vi "DIO 1（Hsot）.vi"() -> ()   [LabVIEW 2019]
uses:
  <vilib>/FPGAPlugInAG/ELVIS III/niLvFpga_Open_ELVIS III.vi
  <vilib>/rvi/interface/common/dynamic/niFpgaDynamicAddResources.vi
  <vilib>/Utility/error.llb/Error Cluster From Error Code.vi
  <vilib>/rvi/errors/niLvFpgaAdjustHostInterfaceError.vi
  <vilib>/FPGAPlugInAG/Dynamic/niLvFpga_Close_Dynamic.vi
  <vilib>/rvi/interface/nirviOpenFPGA/nirviOpenFPGA.xnode
  FPGA Bitfiles/analogio-fpga_FPGATarget_DIO1_c7CcyW3shMY.lvbitx
  DIO 1.vi
  <vilib>/rvi/interface/nirviReadWriteControl/nirviReadWriteControl.xnode
  <vilib>/rvi/interface/nirviCloseFPGA/nirviCloseFPGA.xnode
  NiFpgaLv.dll
  <vilib>/rvi/interface/Simulation/niFpgaSimulationCallBeginRW.vi
panel:
  in  "停止":bool
  out "IN":bool
  in  "OUT":bool
  in  "DIR":bool
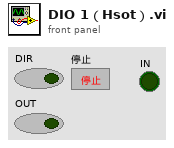
[diagram p1: front panel]
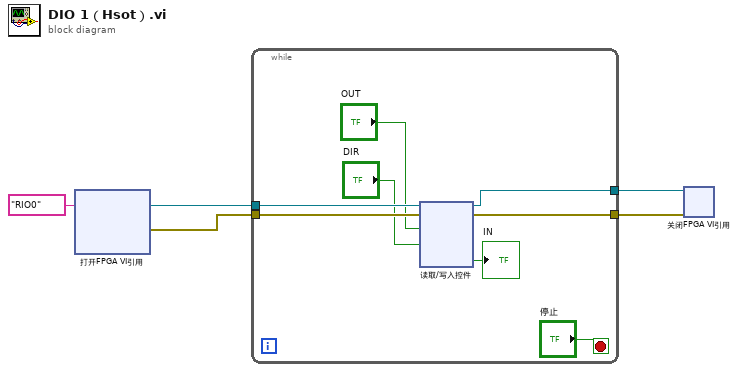
[diagram p0: block diagram]
diagram:
  n1 = xnode "打开FPGA VI引用"("资源名称"=tag "RIO0") -> ("FPGA VI引用输出"=w3:refnum<k20>, "错误输出"=w4:errorcluster)  [unwired: 1 in]
  n2 = while {
    tunnel: w4 -> [w13]
    tunnel: w3 -> [w12]
    tunnel: [w7] -> w2
    tunnel: [w6] -> w1
    stop <- "停止" stop-if-true
    n3 = xnode "读取/写入控件"("FPGA VI引用输入"=w12, "错误输入"=w13, "OUT"="OUT", "DIR"="DIR") -> ("FPGA VI引用输出"=w6:refnum<k20>, "错误输出"=w7:errorcluster, "IN"=→"IN":bool)
  }
  n4 = xnode "关闭FPGA VI引用"("FPGA VI引用输入"=w1, "错误输入"=w2) -> ()  [unwired: 1 out]
